vi "CNR (Multiple).vi"(10 "Array in":T2[](array[typedef]) {"Y" format="%.2f"; "X" format="%.2f"}, 11 "Refnum in":T1) -> (2 "Array out":dbl[](array[numeric]), 3 "Refnum out":T1)   [LabVIEW 2023]
uses:
  <vilib>/vision/Image Controls.llb/IMAQ Image.ctl
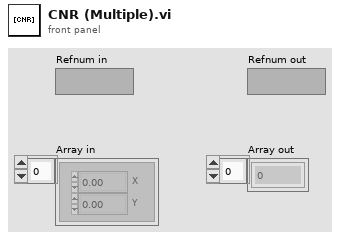
[diagram p1: front panel]
types:
  T1 = typedef "IMAQ Image.ctl" = refnum<image>
  T2 = typedef "IMAQ Point" = cluster{"X":sgl, "Y":sgl}
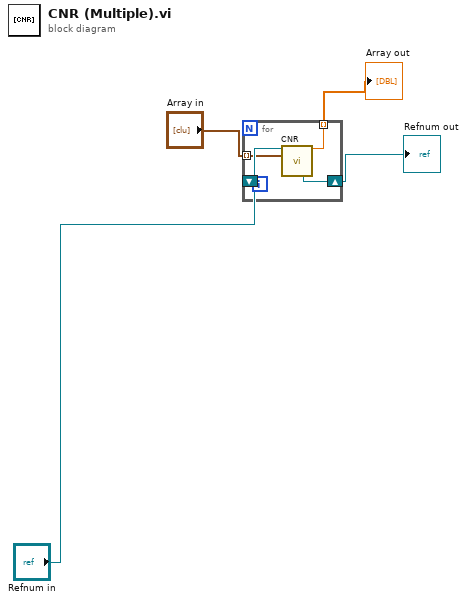
[diagram p0: block diagram]
diagram:
  n1 = for {
    tunnel: [w6] -> w4 mode=indexing
    shift-right: [w7] -> w2
    shift-left: "Refnum in" -> [w8]
    tunnel: "Array in" -> [w5] mode=indexing
    n2 = call "CNR.vi"("Image In"=w8, "Point"=w5) -> ("CNR"=w6:dbl, "Image"=w7:T1)  [unwired: 5 in, 7 out]
  }
  "Array out" <- w4
  "Refnum out" <- w2
